vi "Launch Nested DAQmx Actor.vi"(4 "Debug Alias":string, 6 "Open Actor Core front panel? (F)":bool, 7 "DAQmx Task":refnum<k21>, 8 "error in (no error)":errorcluster, 10 "DAQmx Actor":refnum<class "DAQmx Actor.lvclass">, 11 "Caller Actor in":refnum<class "Actor.lvclass">) -> (0 "error out":errorcluster, 2 "Nested Actor's Enqueuer":refnum<class "Message Enqueuer.lvclass">, 3 "Caller Actor out":refnum<class "Actor.lvclass">)   [LabVIEW 2024]
uses:
  <vilib>/ActorFramework/Actor/Actor.lvclass
  DAQmx Actor.lvclass
  <vilib>/ActorFramework/Message Enqueuer/Message Enqueuer.lvclass
  DAQmx Actor.lvclass/DAQmx Actor.ctl
  C:/Program Files (x86)/National Instruments/LabVIEW 2024/vi.lib/ActorFramework/Actor/Actor.lvclass
  C:/Users/ottoa/OneDrive/Desktop/working copies/DAQmxActor/src/DAQmx Actor/DAQmx Actor/DAQmx Actor.lvclass
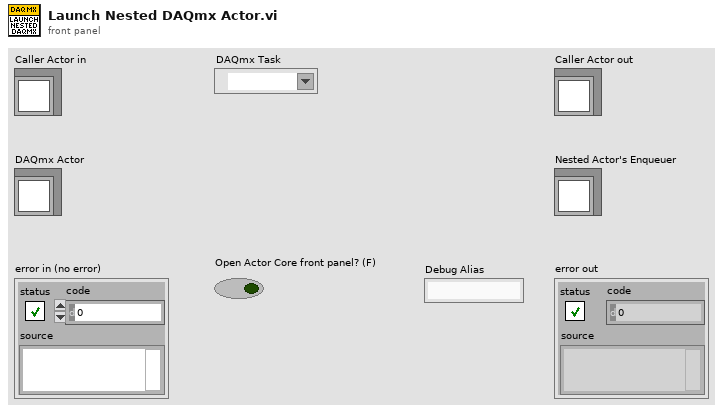
[diagram p1: front panel]
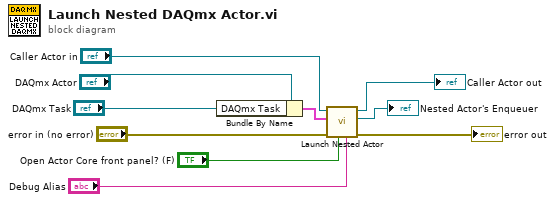
[diagram p0: block diagram]
diagram:
  n1 = Bundle By Name(cluster="DAQmx Actor", "DAQmx Task"="DAQmx Task") -> (w2:cluster{})
  n2 = call <vilib>:"Launch Nested Actor.vi"("Debug Alias"="Debug Alias", "Open Actor Core front panel? (F)"="Open Actor Core front panel? (F)", "error in (no error)"="error in (no error)", "Nested Actor"=w2, "Caller Actor in"="Caller Actor in") -> ("error out"=→"error out":errorcluster, "Nested Actor's Enqueuer"=→"Nested Actor's Enqueuer":refnum<class "Message Enqueuer.lvclass">, "Caller Actor out"=→"Caller Actor out":refnum<class "Actor.lvclass">)  [unwired: 4 in]
